vi "Save Report to File.vi"(8 "error in (no error)":errorcluster, 10 "Report Directory":path, 11 "Report Generator in":refnum<class "Report Generator.lvclass">) -> (0 "error out":errorcluster, 3 "Report Generator out":refnum<class "Report Generator.lvclass">)   [LabVIEW 2020, in "Report Generator.lvclass"]
uses:
  Report Generator.lvclass
  Report Generator.lvclass/Report Generator.ctl
  Report Classes/Test Report/Test Report.lvclass/Test Report.ctl
  Report Classes/Test Report/Test Report.lvclass
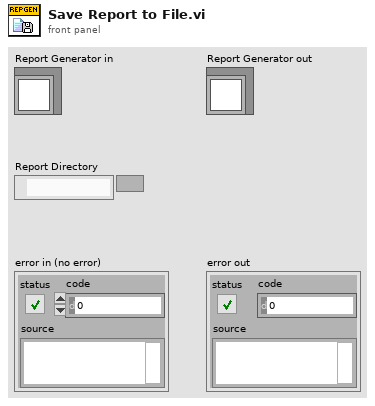
[diagram p1: front panel]
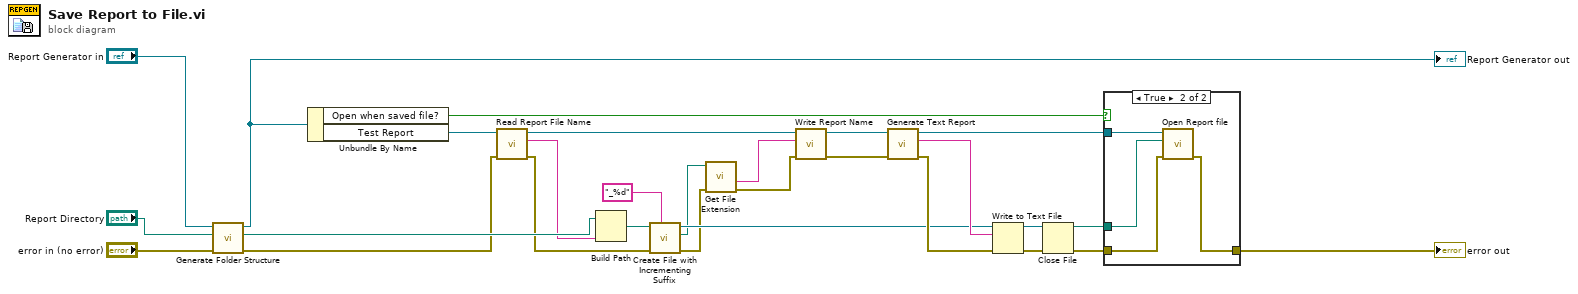
[diagram p0: block diagram]
diagram:
  n1 = call "Generate Folder Structure.vi"("error in (no error)"="error in (no error)", "Report Directory in"="Report Directory", "Report Generator in"="Report Generator in") -> ("error out"=w4:errorcluster, "Report Directory out"=w14:path, "Report Generator out"=w1:refnum<class "Report Generator.lvclass">)  [unwired: 6 in]
  "Report Generator out" <- w1
  n2 = Unbundle By Name(w1) -> ("Open when saved file?"=w5:bool, "Test Report"=w17:refnum<class "Test Report.lvclass">)
  n3 = call-dynamic "Read Report File Name.vi"("error in (no error)"=w4, "Report In"=w17) -> ("error out"=w12:errorcluster, "Report File Name"=w13:string, "Report Out"=w16:refnum<class "Test Report.lvclass">)  [unwired: 6 in, 1 out]
  n4 = Build Path(base path=w14, name or relative path=w13) -> (appended path=w15:path)
  n5 = call <vilib>:"Create File with Incrementing Suffix.vi"("format string (\" (%d)\")"="_%d" ("format string (\" (%d)\")"), "error in (no error)"=w12, "file path"=w15) -> ("error out"=w10:errorcluster, "actual path"=w11:path, "refnum out"=w19:refnum<file>)  [unwired: 6 in]
  n6 = call <vilib>:"Get File Extension.vi"("error in (no error)"=w10, "file"=w11) -> ("error out"=w7:errorcluster, "filename without extension"=w8:string)  [unwired: 5 in, 3 out]
  n7 = call "Write Report Name.vi"("error in (no error)"=w7, "Report Name"=w8, "Report In"=w16) -> ("error out"=w6:errorcluster, "Report Out"=w9:refnum<class "Test Report.lvclass">)  [unwired: 7 in]
  n8 = call-dynamic "Generate Text Report.vi"("error in (no error)"=w6, "Report In"=w9) -> ("error out"=w20:errorcluster, "Text output"=w23:string, "Report Out"=w27:refnum<class "Test Report.lvclass">)  [unwired: 7 in]
  n9 = Write to Text File(file (use dialog)=w19, text=w23, error in=w20) -> (refnum out=w21:refnum<file>, error out=w22:errorcluster)  [unwired: 1 in, 1 out]
  n10 = Close File(refnum=w21, error in=w22) -> (path=w26:path, error out=w24:errorcluster)
  n11 = case shown="True" w5 {
    tunnel: w24 -> [w29 w33]
    tunnel: [w29 w32] -> w25
    tunnel: w26 -> [_ w31]
    tunnel: w27 -> [_ w30]
    frame False {
    }
    frame True {
      n12 = call-dynamic "Open Report file.vi"("error in (no error)"=w33, "Report file path"=w31, "Report In"=w30) -> ("error out"=w32:errorcluster)  [unwired: 7 in, 1 out]
    }
  }
  "error out" <- w25
